vi "Extract RxUDP Header from Buffer.vi"(11 "ReadBuffer in":u8[](array[numeric])) -> (2 "Udp Message":u8[](array[numeric]), 3 "Header":u32[](array[numeric]))   [LabVIEW 2024]
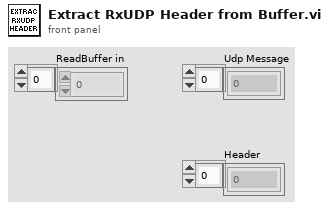
[diagram p1: front panel]
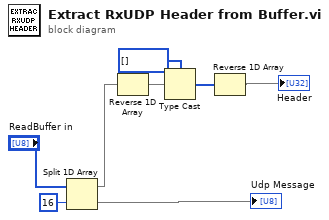
[diagram p0: block diagram]
diagram:
  n1 = Split 1D Array(array="ReadBuffer in", index=16) -> (first subarray=w7:u8[], second subarray=→"Udp Message":u8[])
  n2 = Reverse 1D Array(array=w7) -> (reversed array=w4:u8[])
  n3 = Type Cast(type=u32[] [] ("index"), x=w4) -> (*(type *) &x=w6:u32[])
  n4 = Reverse 1D Array(array=w6) -> (reversed array=→"Header":u32[])
